vi "__VI to Create Object DVR.vi"() -> ()   [LabVIEW 2016, in "SLL Scripting.lvlib" / "SLL Class DVR API Generator.lvlib"]
uses:
  SLL Class DVR API Generator.lvlib
  _Example/My Sample Class.lvclass
panel:
  in  "LabVIEW Object":refnum<class>
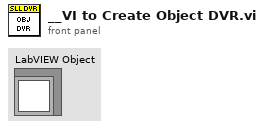
[diagram p1: front panel]
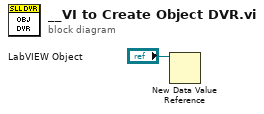
[diagram p0: block diagram]
diagram:
  n1 = New Data Value Reference(data value="LabVIEW Object") -> ()  [unwired: 1 in, 2 out]
